vi "[FGV]Read Template.vi"(10 "Project Name":string, 11 "RootPath":path) -> (0 "error out":errorcluster)   [LabVIEW 2019]
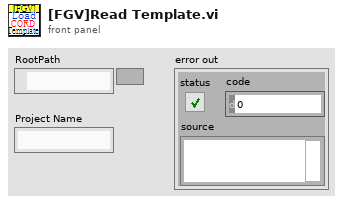
[diagram p1: front panel]
types:
  T1 = typedef "IMAQ Image.ctl" = refnum<image>
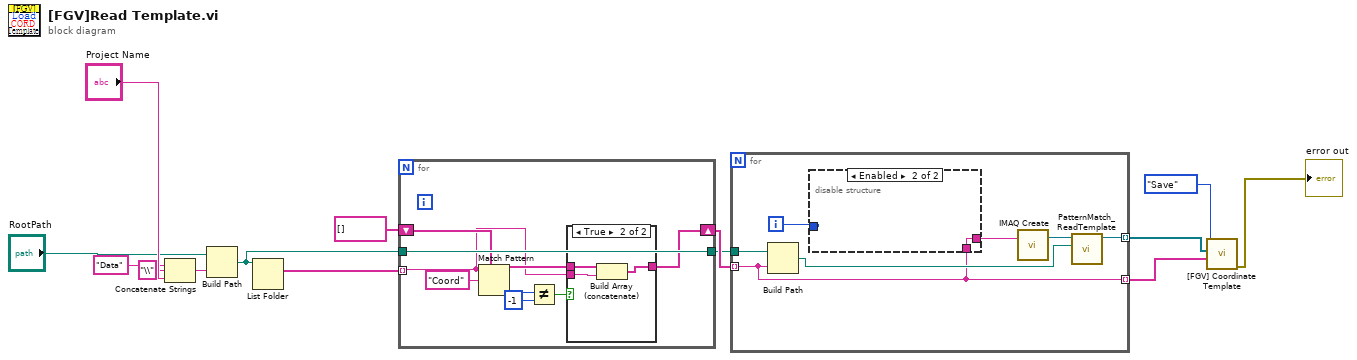
[diagram p0: block diagram]
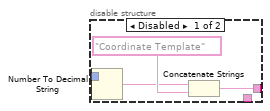
[diagram p2: hidden frame]
diagram:
  n1 = Concatenate Strings("Data" ("string"), "\\" ("string"), "Project Name") -> (w8:string)
  n2 = Build Path(base path="RootPath", name or relative path=w8) -> (appended path=w10:path)
  n3 = List Folder(path=w10) -> (filenames=w9:string[])  [unwired: 3 in, 3 out]
  n4 = for {
    tunnel: w9 -> [w16] mode=indexing
    tunnel: w10 -> [w19]
    tunnel: [w19] -> w3
    shift-right: [w15] -> w4
    shift-left: string[] [] -> [w17]
    n5 = Match Pattern(string=w16, regular expression="Coord") -> (offset past match=w21:i32)  [unwired: 1 in, 3 out]
    n6 = Not Equal?(x=w21, y=-1) -> (x != y?=w18:bool)
    n7 = case shown="True" w18 {
      tunnel: w17 -> [w23 w26]
      tunnel: w16 -> [_ w25]
      tunnel: [w23 w24] -> w15
      frame False {
      }
      frame True {
        n8 = Build Array (concatenate)(w26, w25) -> (w24:string[])
      }
    }
  }
  n9 = for {
    tunnel: w4 -> [w27] mode=indexing
    tunnel: w3 -> [w29]
    tunnel: [w28] -> w2 mode=indexing
    tunnel: [w27] -> w1 mode=indexing
    i -> [w30]
    n10 = Build Path(base path=w29, name or relative path=w27) -> (appended path=w31:path)
    n11 = disable-structure shown="Enabled" {
      disable-tunnel: [w37 w38] -> w32
      disable-tunnel: w30 -> [w34 _]
      disable-tunnel: w27 -> [_ w38]
      frame Disabled {
        n12 = Number To Decimal String(number=w34) -> (decimal integer string=w35:string)  [unwired: 1 in]
        n13 = Concatenate Strings(w35, "Coordinate Template" ("string")) -> (w37:string)
      }
      frame Enabled {
      }
    }
    n14 = call "IMAQ Create"("Image Name"=w32) -> ("New Image"=w33:T1)  [unwired: 4 in, 1 out]
    n15 = call "PatternMatch_ReadTemplate.vi"("template path"=w31, "Template"=w33) -> ("Template Out"=w28:T1)  [unwired: 8 in, 1 out]
  }
  n16 = call "[FGV] Coordinate Template.vi"("Image Name Array"=w1, "Image Array"=w2, "Command"=enum16{"Initialize", "Save", "Read"}."Save") -> ("error out"=→"error out":errorcluster)  [unwired: 6 in, 2 out]
